vi "Set Word Ref.vi"(8 "error in (no error)":errorcluster, 10 "Word Ref":refnum<k24>, 11 "MS-Word in":refnum<class "MS-Word.lvclass">) -> (0 "error out":errorcluster, 3 "MS-Word out":refnum<class "MS-Word.lvclass">)   [LabVIEW 2017, in "LabVIEW NPOI.lvlib" / "MS-Word.lvclass"]
uses:
  MS-Word.lvclass
  C:/Users/Neo/Desktop/Dev_Tools_BR/LabVIEW_NPOI/lib/NPOI 2.1.1/NPOI.OOXML.dll
  lib/NPOI 2.1.1/NPOI.OOXML.dll
  MS-Word.lvclass/MS-Word.ctl
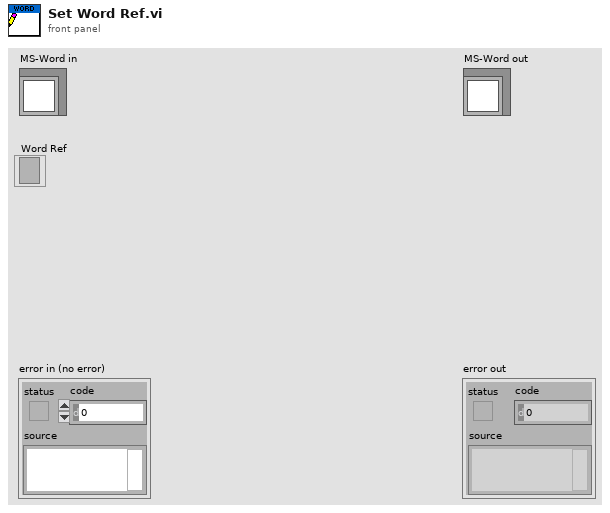
[diagram p1: front panel]
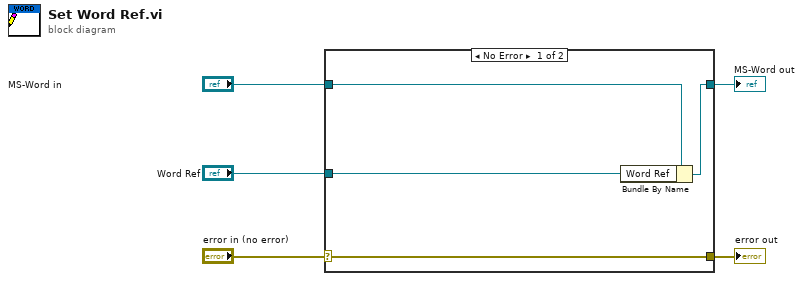
[diagram p0: block diagram]
diagram:
  n1 = case shown="No Error" "error in (no error)" {
    selector: "error in (no error)" -> [w9 w10]
    tunnel: [w9 w10] -> w4
    tunnel: [w7 w11] -> w2
    tunnel: "MS-Word in" -> [w8 w11]
    tunnel: "Word Ref" -> [w6 _]
    frame No Error {
      n2 = Bundle By Name(cluster=w8, "Word Ref"=w6) -> (w7:refnum<class "MS-Word.lvclass">)
    }
    frame Error {
    }
  }
  "error out" <- w4
  "MS-Word out" <- w2
